vi "GlobalCamOpen.vi"() -> ()   [LabVIEW 2010]
panel:
  in  "Camera Opened":u32
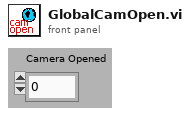
[diagram p1: front panel]
diagram:
